vi "Calculate_CompleteFilePath.vi"(8 "error in":errorcluster, 11 "Process in":refnum<class "Process.lvclass">) -> (0 "error out":errorcluster, 2 "Process Absolute Path":path, 3 "Process out":refnum<class "Process.lvclass">)   [LabVIEW 2013, in "Process.lvclass"]
uses:
  Process.lvclass
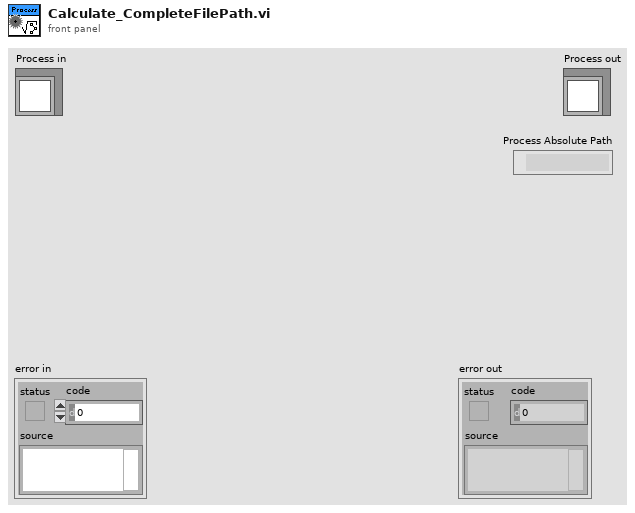
[diagram p1: front panel]
types:
  T1 = typedef "Process.lvclass/EnumProcess.ctl" = enum16{"Message handler", "Template"}
  T2 = typedef "paramsExternalProcesses.ctl" = cluster{"Path":path, "Timeout":dbl, "viInitString":string, "State":enum32{"Invalid", "Standard", "Closed", "Hidden", "Minimized", "Maximized"}}
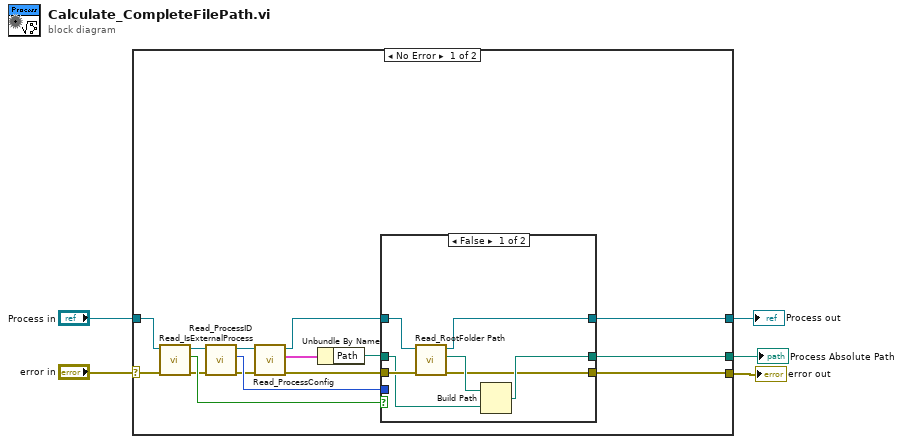
[diagram p0: block diagram]
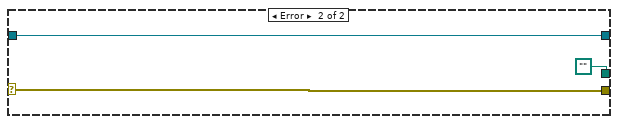
[diagram p3: hidden frame]
diagram:
  n1 = case shown="No Error" "error in" {
    selector: "error in" -> [w12 w33]
    tunnel: [w11 w33] -> w4
    tunnel: [w6 w32] -> w2
    tunnel: "Process in" -> [w10 w32]
    tunnel: [w9 path ""] -> w1
    frame No Error {
      n2 = call-dynamic "Read_IsExternalProcess.vi"("error in (no error)"=w12, "Process in"=w10) -> ("error out"=w14:errorcluster, "ExternalProcess ?"=w18:bool, "Process out"=w15:refnum<class "Process.lvclass">)  [unwired: 7 in]
      n3 = call-dynamic "Read_ProcessID.vi"("error in (no error)"=w14, "Process in"=w15) -> ("error out"=w16:errorcluster, "Process"=w19:T1, "Process out"=w17:refnum<class "Process.lvclass">)  [unwired: 7 in]
      n4 = call-dynamic "Read_ProcessConfig.vi"("error in (no error)"=w16, "Process in"=w17) -> ("error out"=w20:errorcluster, "ProcessConfig"=w8:T2, "Process out"=w7:refnum<class "Process.lvclass">)  [unwired: 7 in]
      n5 = Unbundle By Name(w8) -> ("Path"=w13:path)
      n6 = case shown="False" w18 {
        tunnel: w19 -> [_ _]
        tunnel: [w23 w30] -> w9
        tunnel: w13 -> [w24 w30]
        tunnel: w20 -> [w27 w29]
        tunnel: [w22 w29] -> w11
        tunnel: w7 -> [w26 w28]
        tunnel: [w21 w28] -> w6
        frame False {
          n7 = call-dynamic "Read_RootFolder Path.vi"("error in (no error)"=w27, "Process in"=w26) -> ("error out"=w22:errorcluster, "RootFolder Path"=w25:path, "Process out"=w21:refnum<class "Process.lvclass">)  [unwired: 7 in]
          n8 = Build Path(base path=w25, name or relative path=w24) -> (appended path=w23:path)
        }
        frame True {
        }
      }
    }
    frame Error {
    }
  }
  "error out" <- w4
  "Process out" <- w2
  "Process Absolute Path" <- w1
